vi "Append_tree_files.vi"(2 "Channel Values In":string[][](array[string]), 3 "Accept Array":bool[](array[boolean]), 4 "Filename":path) -> ()   [LabVIEW 2010]
uses:
  Results_plotter_Global.vi
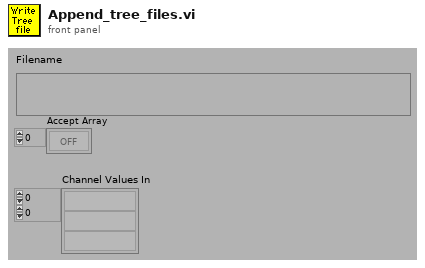
[diagram p1: front panel]
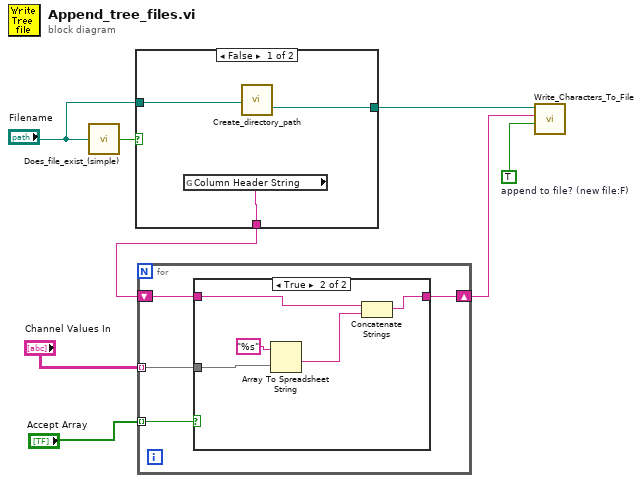
[diagram p0: block diagram]
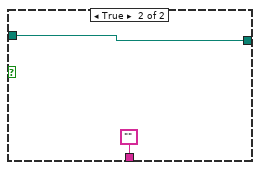
[diagram p2: hidden frame]
diagram:
  w1 = TRUE  # append to file? (new file:F)
  n1 = call "Does_file_exist_(simple).vi"("Pathname"="Filename") -> ("exists?"=w8:bool)
  n2 = case shown="False" w8 {
    tunnel: [w11 ""] -> w7
    tunnel: "Filename" -> [w10 w12]
    tunnel: [w9 w12] -> w2
    frame False {
      n3 = global read "Results_plotter_Global.vi" "Column Header String"() -> (w11:string)
      n4 = call "Create_directory_path.vi"("Path name"=w10) -> ("Path name Out"=w9:path)
    }
    frame True {
    }
  }
  n5 = for {
    shift-right: [w15] -> w3
    shift-left: w7 -> [w14]
    tunnel: "Accept Array" -> [w17] mode=indexing
    tunnel: "Channel Values In" -> [w16] mode=indexing
    n6 = case shown="True" w17 {
      tunnel: w16 -> [_ w23]
      tunnel: [w18 w20] -> w15
      tunnel: w14 -> [w18 w21]
      frame False {
      }
      frame True {
        n7 = Array To Spreadsheet String(array=w23, 3:"%s" ("format string")) -> (spreadsheet string=w19:string)  [unwired: 1 out]
        n8 = Concatenate Strings(w21, w19) -> (w20:string)
      }
    }
  }
  n9 = call "Write_Characters_To_File.vi"("file path (dialog if empty)"=w2, "character string"=w3, "append to file? (new file:F)"=w1) -> ()  [unwired: 2 in, 4 out]
